vi "KE622x -- Get Analog Filter State.vi"(0 "Resource In":refnum<visa-resource-name>, 1 "Check For SCPI Errors? (T)":bool=TRUE, 11 "error in (no error)":errorcluster) -> (4 "Resource Out (dupl)":refnum<visa-resource-name>, 8 "Analog Filter State":T1=enum."On", 15 "error out":errorcluster)   [LabVIEW 2019, in "Keithley 622x.lvlib"]
doc: "Returns the state of the analog output filter on the 622x instrument, either 'On' or 'Off'. If the filter is 'On', the output response speed is decreased."
uses:
  Keithley 622x.lvlib
  Typedefs/KE622x -- On Off Control.ctl
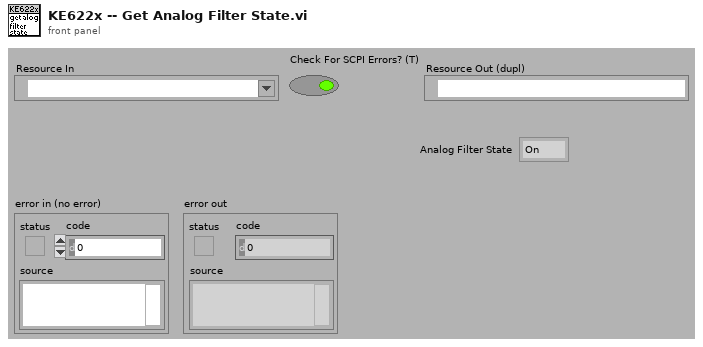
[diagram p1: front panel]
types:
  T1 = typedef "Keithley 622x.lvlib/KE622x -- On Off Control.ctl" = enum16{"Off", "On"}
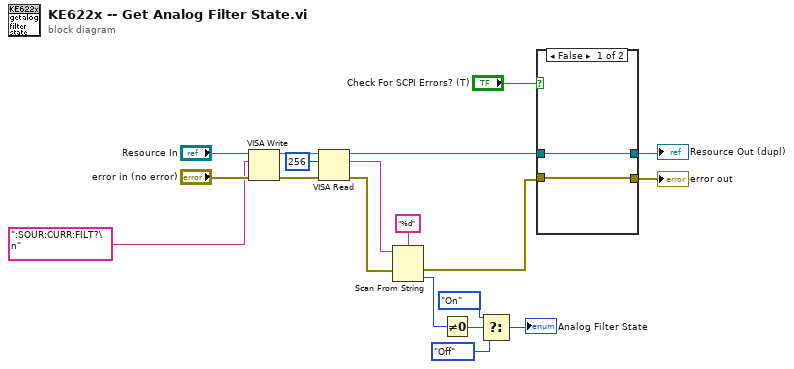
[diagram p0: block diagram]
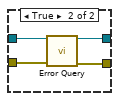
[diagram p2: hidden frame]
diagram:
  n1 = VISA Write(VISA resource name="Resource In", write buffer=":SOUR:CURR:FILT?\n" ("format string"), error in (no error)="error in (no error)") -> (VISA resource name out=w13:refnum<visa-resource-name>, error out=w12:errorcluster)  [unwired: 1 out]
  n2 = VISA Read(VISA resource name=w13, byte count=u32 256, error in (no error)=w12) -> (VISA resource name out=w6:refnum<visa-resource-name>, read buffer=w8:string, error out=w10:errorcluster)  [unwired: 1 out]
  n3 = Scan From String(format string="%d", input string=w8, error in=w10) -> (error out=w7:errorcluster, output 1=w5:i32)  [unwired: 2 in, 2 out]
  n4 = Not Equal To 0?(x=w5) -> (x != 0?=w4:bool)
  n5 = Select(t=KE622x_--_On_Off_Control."On" ("Analog Filter State"), s=w4, f=KE622x_--_On_Off_Control."Off") -> (s? t:f=→"Analog Filter State":T1)
  n6 = case shown="False" "Check For SCPI Errors? (T)" {
    tunnel: w6 -> [w21 w25]
    tunnel: w7 -> [w20 w24]
    tunnel: [w20 w23] -> w15
    tunnel: [w21 w22] -> w16
    frame False {
    }
    frame True {
      n7 = call "Error Query.vi"("VISA Resource In"=w25, "error in (no error)"=w24) -> ("VISA Resource Out (dupl)"=w22:refnum<visa-resource-name>, "error out"=w23:errorcluster)  [unwired: 10 in, 2 out]
    }
  }
  "Resource Out (dupl)" <- w16
  "error out" <- w15
